vi "subBuildSingleTarget.vi"(8 "error in (no error)":errorcluster, 9 "Target":string="My Computer", 10 "Build Spec":string, 11 "Project":path) -> (0 "error out":errorcluster, 1 "Output Message":string, 2 "Exit Code (0)":i32)   [LabVIEW 2016, in "lvcommonbuild.lvlib"]
uses:
  lvcommonbuild.lvlib
  <vilib>/Utility/error.llb/DialogType.ctl
  <vilib>/AppBuilder/AB_API_Simple/Build (path).vi
  <vilib>/AppBuilder/AB_API_Simple/NI_App_Builder_API.lvlib
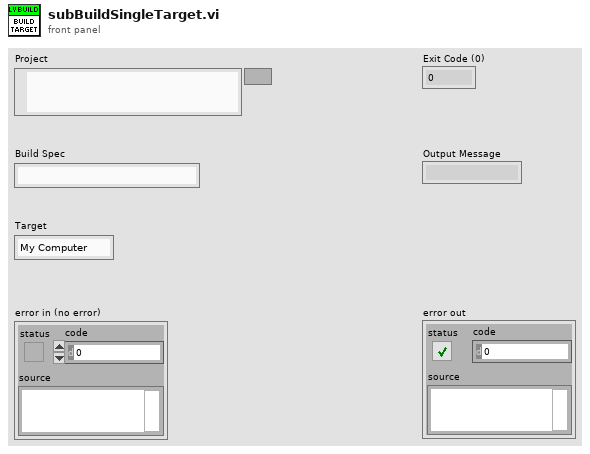
[diagram p1: front panel]
types:
  T1 = typedef "DialogType.ctl" = u16
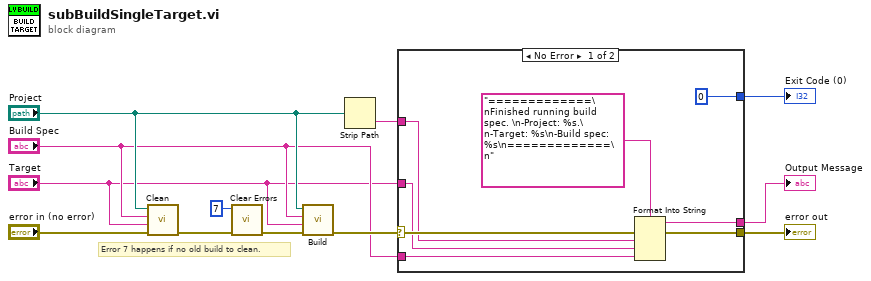
[diagram p0: block diagram]
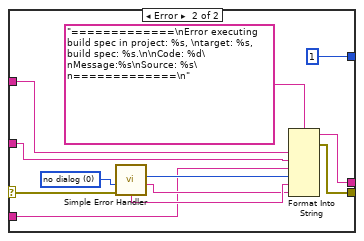
[diagram p2: hidden frame]
diagram:
  # "Error 7 happens if no old build to clean."
  n1 = call <vilib>:"Clean.vi"("error in (no error)"="error in (no error)", "Name of target (My Computer)"="Target", "Name of build specification (if empty: clean all)"="Build Spec", "Path to project"="Project") -> ("error out"=w12:errorcluster)  [unwired: 7 in]
  n2 = call <vilib>:"Clear Errors.vi"("error in (no error)"=w12, "specific error code to clear (0: all)"=7) -> ("error out"=w11:errorcluster)  [unwired: 4 in, 1 out]
  n3 = call-poly <vilib>:"Build.vi"("error in (no error)"=w11, "Name of target (My Computer)"="Target", "Name of build specification (if empty: build all)"="Build Spec", "Path to project"="Project") -> ("error out"=w9:errorcluster)  [unwired: 6 in, 1 out]
  n4 = Strip Path(path="Project") -> (name=w8:string)  [unwired: 1 out]
  n5 = case shown="No Error" w9 {
    selector: w9 -> [w19 w31]
    tunnel: w8 -> [w18 w24]
    tunnel: "Target" -> [w17 w23]
    tunnel: [w16 w32] -> w2
    tunnel: [0 ("Exit Code (0)") 1 ("Exit Code (0)")] -> w1
    tunnel: "Build Spec" -> [w14 w22]
    tunnel: [w13 w21] -> w3
    frame No Error {
      n6 = Format Into String(format string="=============\nFinished running build spec. \n-Project: %s.\n-Target: %s\n-Build spec: %s\n=============\n", error in=w19, w18, w17, w14) -> (resulting string=w16:string, error out=w13:errorcluster)  [unwired: 1 in]
    }
    frame Error {
      w30 = T1 0 items=["no dialog", "OK message", "continue or stop message", "OK message + warnings", "continue/stop + warnings"] ("type of dialog (OK msg:1)")
      n7 = call <vilib>:"Simple Error Handler.vi"("type of dialog (OK msg:1)"=w30, "error in (no error)"=w31) -> ("code out"=w25:i32, "source out"=w26:string, "message"=w27:string)  [unwired: 3 in, 2 out]
      n8 = Format Into String(format string="=============\nError executing build spec in project: %s, \ntarget: %s, build spec: %s.\n\nCode: %d\nMessage:%s\nSource: %s\n=============\n", w24, w23, w22, w25, w27, w26) -> (resulting string=w32:string, error out=w21:errorcluster)  [unwired: 2 in]
    }
  }
  "error out" <- w3
  "Output Message" <- w2
  "Exit Code (0)" <- w1
